vi "O2 Leaktest Test.vi"(6 "Aktion":T1, 8 "O2":sgl caption="%" format="%.3f", 9 "Status":string) -> (0 "countdown":dbl, 1 "Status":string, 2 "Fertig?":bool, 3 "Messgasdruck":sgl, 4 "Aktion":T1)   [LabVIEW 2020, in "O2 Dichtheitstest.lvlib"]
uses:
  O2 Dichtheitstest.lvlib
  Aktion O2 Test.ctl
  Amium PNS/Aktion FGV Amium Daten.ctl
  Seiten/CalGas Aufschaltung/FGV CalGas Aktionen.ctl
  Aktion FGV O2 Leak.ctl
  Seiten/CalGas Aufschaltung/Auswahl Analysator.ctl
  Seiten/FT-IR/FGV FT-IR Gasliste Aktionen.ctl
  Sprachverwaltung/FGV Aktion Tabelle zerlegen.ctl
  Funktionstasten/Funktionstasten-Aktion.ctl
  Funktionstasten/Zustaende.ctl
  Seiten/CalGas Aufschaltung/CalGas Aufschaltung.lvlib
  Funktionstasten/Funktionstasten.lvlib
  Seiten/FT-IR/FT-IR.lvlib
  Sprachverwaltung/Sprachverwaltung.lvlib
  Amium PNS/Amium PNS.lvlib
  Linearisierung V2/Linearisierung v2.lvlib
  Allgemein/allgemeine Sub-VIs.lvlib
  Messdaten/Messdaten.lvlib
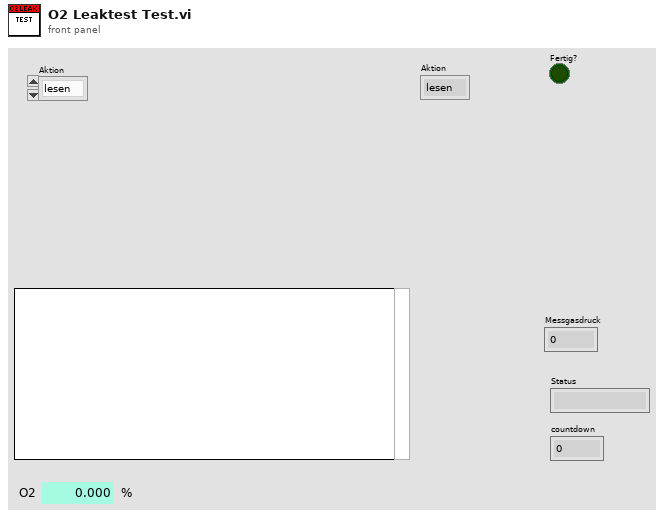
[diagram p1: front panel]
types:
  T1 = typedef "O2 Dichtheitstest.lvlib/Aktion O2 Test.ctl" = enum16{"lesen", "ini", "0-Gas", "Auswerten", "Fertig"}
  T2 = typedef "Amium PNS.lvlib/Aktion FGV Amium Daten.ctl" = enum16{"lesen", "Komm Daten", "Daten", "Error", "Regler", "Grenzwerte", "laden", "speichern"}
  T3 = typedef "Sprachverwaltung.lvlib/FGV Aktion Tabelle zerlegen.ctl" = enum16{"laden", "vereinzeln", "speichern"}
  T4 = typedef "FT-IR.lvlib/FGV FT-IR Gasliste Aktionen.ctl" = enum16{"lesen", "Gasliste FT-IR", "Gasliste ausgelesen", "laden", "speichern", "löschen"}
  T5 = typedef "CalGas Aufschaltung.lvlib/Auswahl Analysator.ctl" = enum16{"FT-IR", "FID", "PMA", "PMA/FID/FT-IR"}
  T6 = typedef "O2 Dichtheitstest.lvlib/Aktion FGV O2 Leak.ctl" = enum16{"lesen", "O2 settings", "Pfad", "Protokoll", "laden", "speichern"}
  T7 = typedef "CalGas Aufschaltung.lvlib/FGV CalGas Aktionen.ctl" = enum16{"lesen", "Analysator Auswahl", "Def.CalGas", "Aufschaltung CalGas", "laden", "speichern", "KAL extrahieren"}
  T8 = typedef "Funktionstasten.lvlib/Zustaende.ctl" = enum16{"Standby", "Pause", "Eco", "Messen", "Kalibrieren", "Spülen Filter", "Spülen Leitung", "Umgebungsluft", "0-Gas", "Cal-Gas", "CG zu PNS", "-------------", "Init 1", "Init 2", "Init 3", "Init 4", "Messen vorbereiten", "Messen durchführen", "Exit"}
  T9 = typedef "Funktionstasten.lvlib/Funktionstasten-Aktion.ctl" = enum16{"Initialisieren", "Zustand setzen", "Taste gedrückt", "Fehler speichern", "Lesen", "Manuell", "Remote", "Bitparallel", "Samplepoint", "Zeit Prüfen", "reset Umschalten"}
  T10 = typedef "Amium PNS.lvlib/Daten Cluster.ctl" = cluster{"Amium Zustände":T11, "Samplepoint am PNS":i16, "Gerätekennung":string, "aktiver Samplepoint":i16[], "Messgasdruck":sgl}
  T11 = typedef "Amium PNS.lvlib/Amium Zustand.ctl" = u16
  T12 = typedef "O2 Dichtheitstest.lvlib/O2 Settings.ctl" = cluster{"Kalibriergas":T13, "Aufschaltpunkt":T13, "Nullgas Aufschaltzeit:":sgl, "Datenerfassungszeit:":sgl, "Grenzwert: O2":sgl, "Grenzwert: Messgasdruck":sgl, "Grenzwert: Messgasdruck 2":sgl}
  T13 = typedef "Auswahlfeld.ctl" = u16
  T14 = typedef "CalGas Aufschaltung.lvlib/Aufschaltung CalGas.ctl" = cluster{"Kalibriergas":T13, "Aufschaltpunkt":T15, "Analysator":T5}
  T15 = typedef "CalGas Aufschaltung.lvlib/Auswahl Aufschaltpunkt.ctl" = enum16{"über Filterblock", "Analysator direkt", "über PNS", "Entnahme", "Gasdivider"}
  T16 = typedef "Zahlen-Eingabefeld.ctl" = sgl
  T17 = typedef "String - Ausgabefeld.ctl" = string
  T18 = typedef "O2 Dichtheitstest.lvlib/Protokoll LeakTest.ctl" = cluster{"O2":sgl, "Messgasdruck":sgl, "Startzeit":timestamp, "Endzeit":timestamp, "Bestanden?":bool}
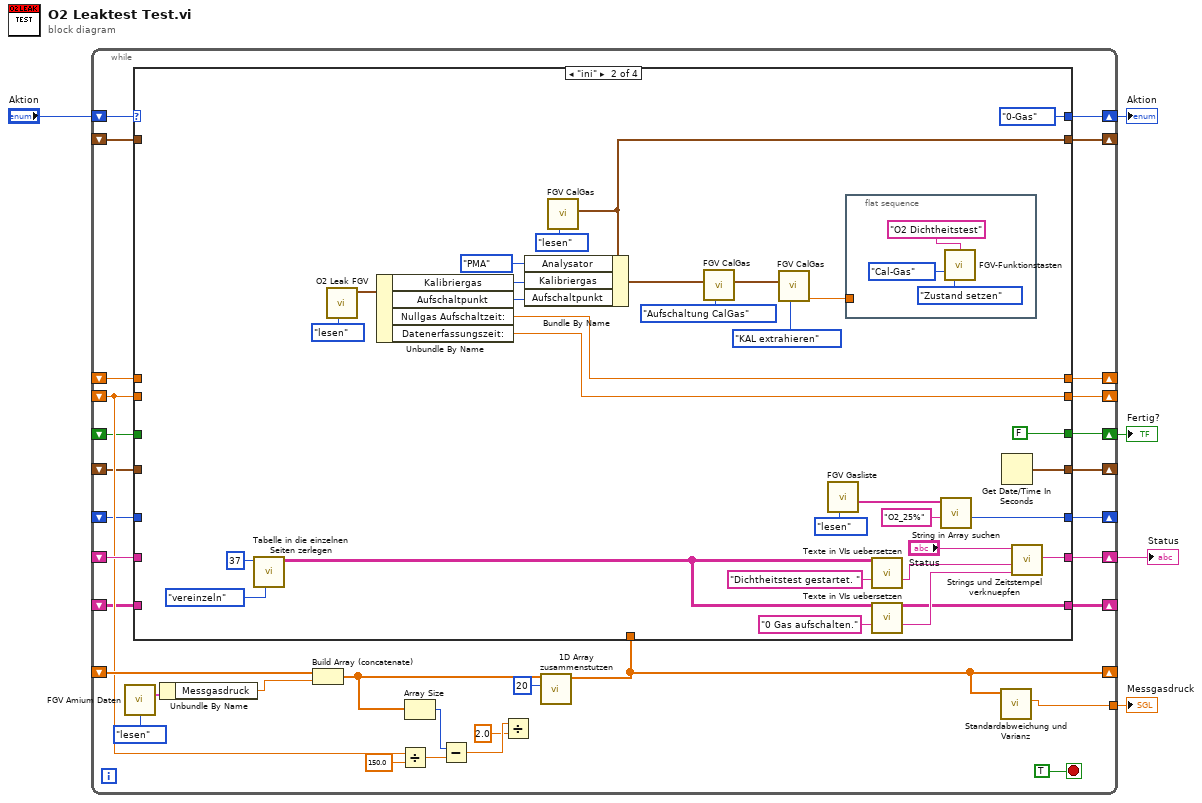
[diagram p0: block diagram]
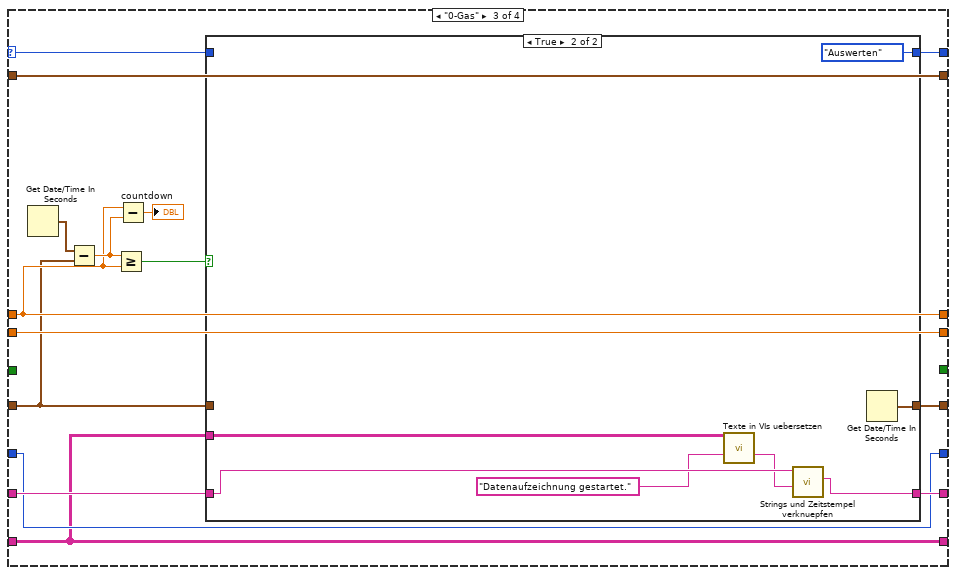
[diagram p3: hidden frame]
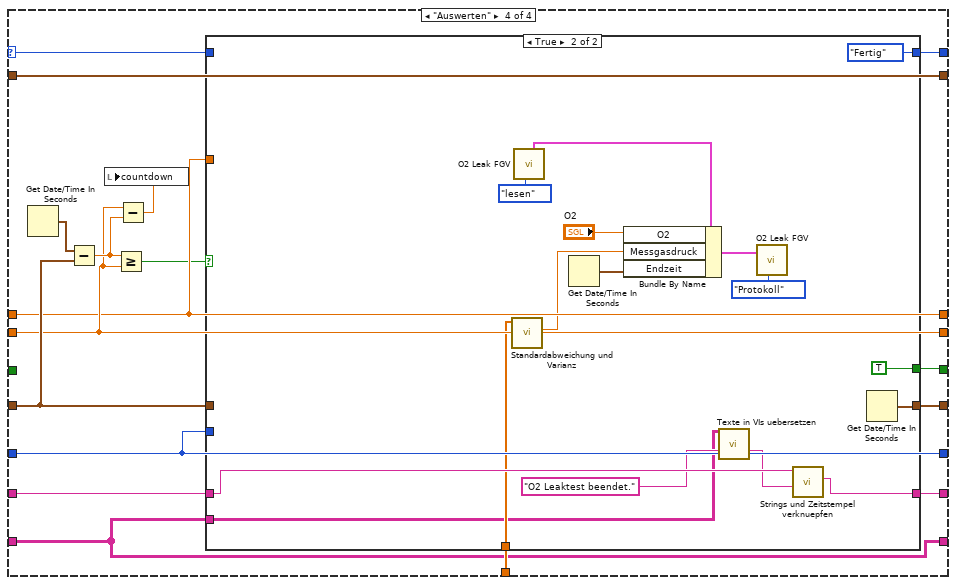
[diagram p5: hidden frame]
diagram:
  n1 = while {
    shift-right: [w35] -> w3
    shift-left: "Aktion" -> [w36]
    shift-right: [w34] -> _
    shift-left: _ -> [w33]
    shift-right: [w32] -> w4
    shift-left: _ -> [w31]
    shift-right: [w11] -> _
    shift-left: _ -> [w22]
    shift-right: [w21] -> _
    shift-left: _ -> [w16]
    shift-right: [w20] -> _
    shift-left: _ -> [w19]
    shift-right: [w18] -> w2
    shift-left: _ -> [w17]
    shift-right: [w15] -> _
    shift-left: _ -> [w14]
    shift-right: [w13] -> _
    shift-left: _ -> [w12]
    tunnel: [w10] -> w1
    shift-right: [w6] -> _
    shift-left: _ -> [w7]
    stop <- TRUE stop-if-true
    n2 = call "FGV Amium Daten.vi"("Aktion"=Aktion_FGV_Amium_Daten."lesen") -> ("Amium Daten"=w23:T10)  [unwired: 9 in, 5 out]
    n3 = Unbundle By Name(w23) -> ("Messgasdruck"=w25:sgl)
    n4 = Build Array (concatenate)(w22, w25) -> (w28:sgl[])
    n5 = Divide(x=w19, y=sgl 150.0) -> (x/y=w27:sgl)
    n6 = Array Size(array=w28) -> (size(s)=w26:i32)
    n7 = Subtract(x=w26, y=w27) -> (x-y=w30:sgl)
    n8 = Divide(x=w30, y=sgl 2.0 ("x")) -> ()  [unwired: 1 out]
    n9 = call "1D Array zusammenstutzen.vi"("Anzahl Elemente"=20, "Messdaten"=w28) -> ("Messdaten"=w11:sgl[])  [unwired: 8 in, 1 out]
    n10 = case shown="\"ini\"" w36 {
      selector: w36 -> [w46 _ w90 w119]
      tunnel: [w46 Aktion_O2_Test."0-Gas" ("Aktion") w91 w120] -> w35
      tunnel: [w45 w66 w89 w118] -> w34
      tunnel: w33 -> [w45 _ w89 w118]
      tunnel: [w40 w60 w85 w116] -> w32
      tunnel: w31 -> [w40 _ w86 w117]
      tunnel: [w44 w58 w87 w109] -> w21
      tunnel: [w43 w57 w88 w113] -> w20
      tunnel: w16 -> [w44 _ w87 w109]
      tunnel: w19 -> [w43 _ w88 w113]
      tunnel: [w42 FALSE _ w111] -> w18
      tunnel: w17 -> [w42 _ _ _]
      tunnel: [w41 w55 w83 w114] -> w15
      tunnel: w14 -> [w41 _ w84 w115]
      tunnel: [w39 w51 w82 w110] -> w13
      tunnel: w12 -> [w39 _ w82 w110]
      tunnel: w11 -> [_ _ _ w108]
      tunnel: w7 -> [w38 _ w81 w106]
      tunnel: [w38 w50 w81 w106] -> w6
      frame "lesen", Default {
      }
      frame "ini" {
        n11 = call "Tabelle in die einzelnen Seiten zerlegen.vi"("Aktion"=FGV_Aktion_Tabelle_zerlegen."vereinzeln", "Index (Seite)"=37) -> ("Sprachliste"=w47:string[][])  [unwired: 7 in, 2 out]
        n12 = call "O2 Leak FGV.vi"("Aktion"=Aktion_FGV_O2_Leak."lesen") -> ("O2 Settings"=w70:T12)  [unwired: 6 in, 4 out]
        n13 = Unbundle By Name(w70) -> ("Kalibriergas"=w68:T13, "Aufschaltpunkt"=w67:T13, "Nullgas Aufschaltzeit:"=w58:sgl, "Datenerfassungszeit:"=w57:sgl)
        n14 = call "FGV CalGas.vi"("Aktionen"=FGV_CalGas_Aktionen."lesen") -> ("Aufschaltung CalGas"=w66:T14)  [unwired: 6 in, 4 out]
        n15 = Bundle By Name(cluster=w66, "Analysator"=Auswahl_Analysator."PMA", "Kalibriergas"=w68, "Aufschaltpunkt"=w67) -> (w74:T14)
        n16 = call "FGV CalGas.vi"("Aktionen"=FGV_CalGas_Aktionen."Aufschaltung CalGas", "Aufschaltung CalGas"=w74) -> ("Aufschaltung CalGas"=w76:T14)  [unwired: 5 in, 4 out]
        n17 = call "FGV CalGas.vi"("Aktionen"=FGV_CalGas_Aktionen."KAL extrahieren", "Aufschaltung CalGas"=w76) -> ("Konzentration 2"=w72:T16)  [unwired: 5 in, 4 out]
        n18 = call "FGV Gasliste.vi"("Aktionen"=FGV_FT-IR_Gasliste_Aktionen."lesen") -> ("Aktuelle Gasliste gesamt"=w52:T17[])  [unwired: 8 in, 2 out]
        n19 = flat-sequence {
          tunnel: w72 -> [_]
          frame #0 {
            n20 = call "FGV-Funktionstasten.vi"("Herkunft"="O2 Dichtheitstest", "Zustand"=Zustaende."Cal-Gas", "Aktion"=Funktionstasten-Aktion."Zustand setzen") -> ()  [unwired: 5 in, 8 out]
          }
        }
        n21 = call "Texte in VIs uebersetzen.vi"("Sprachliste"=w47, "String zum Übersetzen"="Dichtheitstest gestartet. ") -> ("String zum Übersetzen"=w62:string)  [unwired: 9 in, 4 out]
        n22 = call "Texte in VIs uebersetzen.vi"("Sprachliste"=w47, "String zum Übersetzen"="0 Gas aufschalten.") -> ("Sprachliste out"=w50:string[][], "String zum Übersetzen"=w64:string)  [unwired: 9 in, 3 out]
        n23 = call "String in Array suchen.vi"("Nach String/Zeichen suchen (-)"="O2_25%", "String-Array"=w52) -> ("Index"=w51:i32)  [unwired: 7 in, 2 out]
        n24 = Get Date/Time In Seconds() -> (seconds since 1Jan1904=w55:timestamp)
        n25 = call "Strings und Zeitstempel verknuepfen.vi"("String 2 hinzufügen"=w64, "String 1 hinzufügen"=w62, "Eingagns String"="Status") -> ("Verknüpfter String"=w60:string)  [unwired: 8 in]
      }
      frame "0-Gas" {
        n26 = Get Date/Time In Seconds() -> (seconds since 1Jan1904=w93:timestamp)
        n27 = Subtract(x=w93, y=w84) -> (x-y=w94:dbl)
        n28 = Greater Or Equal?(x=w94, y=w87) -> (x >= y?=w92:bool)
        n29 = Subtract(x=w87, y=w94) -> (x-y=→"countdown":dbl)
        n30 = case shown="True" w92 {
          tunnel: [w98 Aktion_O2_Test."Auswerten" ("Aktion")] -> w91
          tunnel: w90 -> [w98 _]
          tunnel: w86 -> [w97 w103]
          tunnel: [w97 w102] -> w85
          tunnel: w84 -> [w96 _]
          tunnel: [w96 w104] -> w83
          tunnel: w81 -> [_ w99]
          frame False {
          }
          frame True {
            n31 = call "Texte in VIs uebersetzen.vi"("Sprachliste"=w99, "String zum Übersetzen"="Datenaufzeichnung gestartet." ("String 1 hinzufügen")) -> ("String zum Übersetzen"=w100:string)  [unwired: 9 in, 4 out]
            n32 = call "Strings und Zeitstempel verknuepfen.vi"("String 1 hinzufügen"=w100, "Eingagns String"=w103) -> ("Verknüpfter String"=w102:string)  [unwired: 9 in]
            n33 = Get Date/Time In Seconds() -> (seconds since 1Jan1904=w104:timestamp)
          }
        }
      }
      frame "Auswerten" {
        n34 = Get Date/Time In Seconds() -> (seconds since 1Jan1904=w121:timestamp)
        n35 = Subtract(x=w121, y=w115) -> (x-y=w122:dbl)
        n36 = Greater Or Equal?(x=w122, y=w113) -> (x >= y?=w107:bool)
        n37 = Subtract(x=w113, y=w122) -> (x-y=w112:dbl)
        n38 = local write "countdown"(w112) -> ()
        n39 = case shown="True" w107 {
          tunnel: [w125 Aktion_O2_Test."Fertig" ("Aktion")] -> w120
          tunnel: w119 -> [w125 _]
          tunnel: w117 -> [w124 w139]
          tunnel: [w124 w138] -> w116
          tunnel: w115 -> [w123 _]
          tunnel: [w123 w140] -> w114
          tunnel: [_ TRUE] -> w111
          tunnel: w110 -> [_ _]
          tunnel: w109 -> [_ _]
          tunnel: w108 -> [_ w132]
          tunnel: w106 -> [_ w126]
          frame False {
          }
          frame True {
            n40 = call "Standardabweichung und Varianz.vi"("X"=w132) -> ("Mittelwert"=w131:sgl)  [unwired: 8 in, 2 out]
            n41 = call "O2 Leak FGV.vi"("Aktion"=Aktion_FGV_O2_Leak."lesen") -> ("Protokoll"=w135:T18)  [unwired: 6 in, 4 out]
            n42 = Get Date/Time In Seconds() -> (seconds since 1Jan1904=w130:timestamp)
            n43 = Bundle By Name(cluster=w135, "O2"="O2", "Messgasdruck"=w131, "Endzeit"=w130) -> (w133:T18)
            n44 = call "Texte in VIs uebersetzen.vi"("Sprachliste"=w126, "String zum Übersetzen"="O2 Leaktest beendet." ("String 1 hinzufügen")) -> ("String zum Übersetzen"=w127:string)  [unwired: 9 in, 4 out]
            n45 = call "O2 Leak FGV.vi"("Aktion"=Aktion_FGV_O2_Leak."Protokoll", "Protokoll"=w133) -> ()  [unwired: 5 in, 5 out]
            n46 = call "Strings und Zeitstempel verknuepfen.vi"("String 1 hinzufügen"=w127, "Eingagns String"=w139) -> ("Verknüpfter String"=w138:string)  [unwired: 9 in]
            n47 = Get Date/Time In Seconds() -> (seconds since 1Jan1904=w140:timestamp)
          }
        }
      }
    }
    n48 = call "Standardabweichung und Varianz.vi"("X"=w11) -> ("Mittelwert"=w10:sgl)  [unwired: 8 in, 2 out]
  }
  "Status" <- w4
  "Aktion" <- w3
  "Fertig?" <- w2
  "Messgasdruck" <- w1
